vi "Extract_Province_Data.vi"(8 "Province":string, 11 "Country Data In":string[][](array[string])) -> (3 "Province Data Out":string[][](array[string]))   [LabVIEW 2015]
doc: "This VI extracts the data by province or states. A lot of these rows of data were deprecated from the file by JHU/CSSE on March 21, 2020"
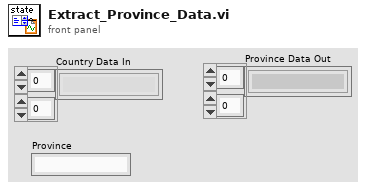
[diagram p1: front panel]
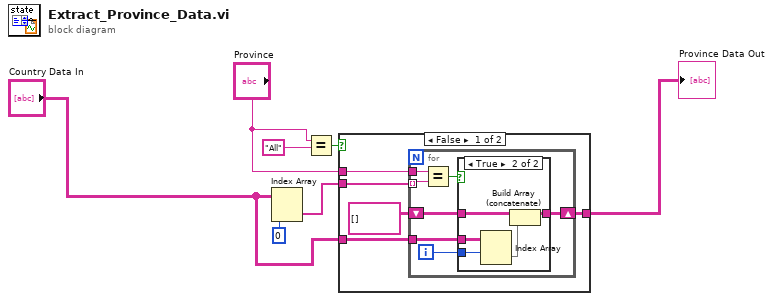
[diagram p0: block diagram]
diagram:
  n1 = Index Array(array="Country Data In", index (col)=0 ("index (row)")) -> (element=w6:string[])  [unwired: 1 in]
  n2 = Equal?(x="Province", y="All") -> (x = y?=w1:bool)
  n3 = case shown="False" w1 {
    tunnel: w6 -> [w12 _]
    tunnel: "Province" -> [w11 _]
    tunnel: "Country Data In" -> [w10 w26]
    tunnel: [w8 w26] -> w3
    frame False {
      n4 = for {
        tunnel: w12 -> [w17] mode=indexing
        tunnel: w11 -> [w19]
        shift-right: [w16] -> w8
        shift-left: string[][] [] -> [w15]
        tunnel: w10 -> [w14]
        i -> [w13]
        n5 = Equal?(x=w19, y=w17) -> (x = y?=w18:bool)
        n6 = case shown="True" w18 {
          tunnel: w15 -> [w20 w25]
          tunnel: [w20 w24] -> w16
          tunnel: w14 -> [_ w23]
          tunnel: w13 -> [_ w22]
          frame False {
          }
          frame True {
            n7 = Index Array(array=w23, index (row)=w22) -> (element=w21:string[])  [unwired: 1 in]
            n8 = Build Array (concatenate)(w25, w21) -> (w24:string[][])
          }
        }
      }
    }
    frame True {
      # "all countries selected"
    }
  }
  "Province Data Out" <- w3
